vi "SSH_command.vi"(7 "password":string, 8 "error in":errorcluster, 9 "Username":string, 10 "Host":string="130.64.87.197", 11 "Command(s) to Execute":string="pwd") -> (0 "error out":errorcluster, 2 "standard error":string, 3 "standard output":string)   [LabVIEW 2012]
panel:
  out "command line input":string
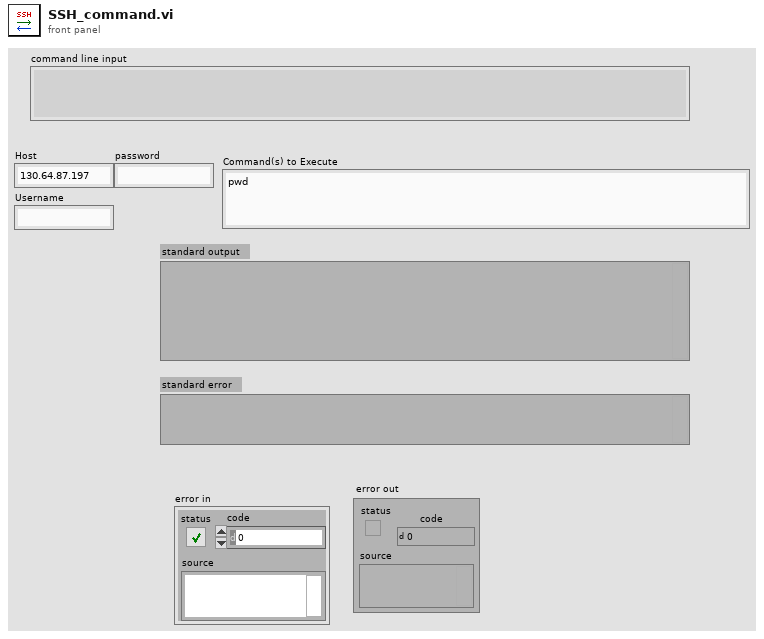
[diagram p1: front panel]
types:
  T1 = enum16{"open", "replace", "create", "open or create", "replace or create", "replace or create with confirmation"}
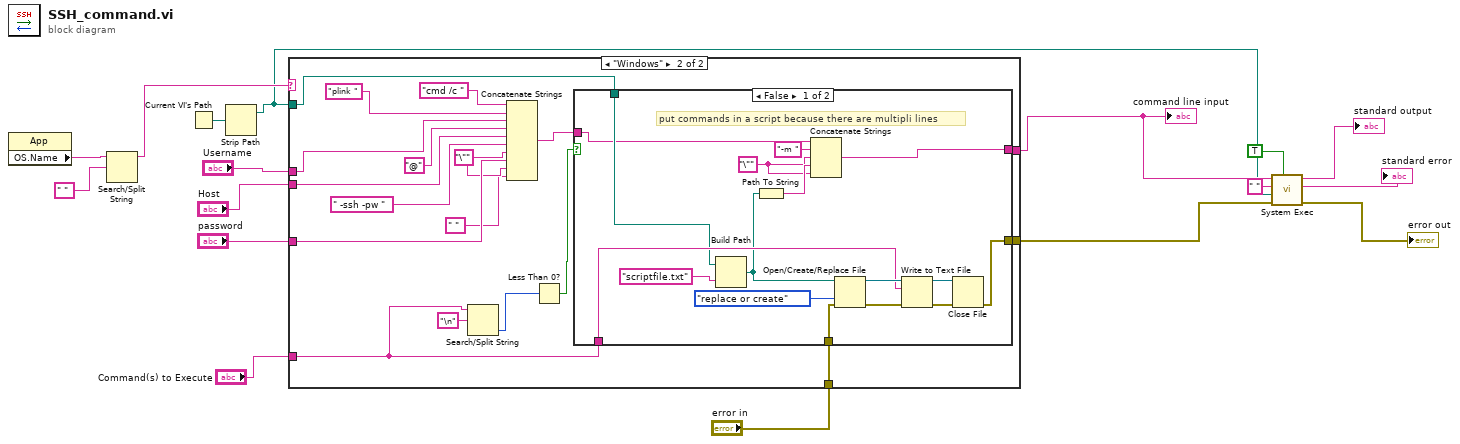
[diagram p0: block diagram]
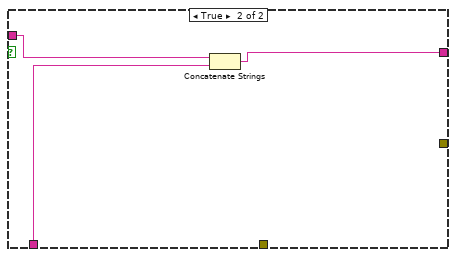
[diagram p3: hidden frame]
diagram:
  n1 = property class="App"() -> ("OS.Name"=w14:string)  [unwired: 2 in, 2 out]
  n2 = Search/Split String(string=w14, search string/char (-)=" ") -> (substring before match=w13:string)  [unwired: 1 in, 2 out]
  n3 = Current VI's Path() -> (path=w17:path)
  n4 = Strip Path(path=w17) -> (stripped path=w7:path)  [unwired: 1 out]
  n5 = case shown="\"Windows\"" w13 {
    tunnel: w7 -> [_ w30]
    tunnel: "Username" -> [_ w34]
    tunnel: "Host" -> [_ w32]
    tunnel: "password" -> [_ w27]
    tunnel: "Command(s) to Execute" -> [_ w22]
    tunnel: [_ w28] -> w10
    tunnel: [_ w19] -> w2
    tunnel: "error in" -> [_ w18]
    frame "False", Default {
    }
    frame "Windows" {
      w26 = "\"" ("string")
      n6 = Search/Split String(string=w22, search string/char (-)="\n") -> (offset of match=w21:i32)  [unwired: 1 in, 2 out]
      n7 = Concatenate Strings("cmd /c " ("string"), "plink " ("name or relative path"), w34, "@" ("string"), w32, " -ssh -pw " ("string"), w26, w27, w26, " " ("string")) -> (w29:string)
      n8 = Less Than 0?(x=w21) -> (x < 0?=w20:bool)
      n9 = case shown="False" w20 {
        tunnel: w22 -> [w46 w53]
        tunnel: w30 -> [w44 _]
        tunnel: w29 -> [w43 w54]
        tunnel: [w40 w52] -> w28
        tunnel: [w37 _] -> w19
        tunnel: w18 -> [w36 _]
        frame False {
          w38 = "\"" ("string")
          # "put commands in a script because there are multipli lines"
          n10 = Build Path(base path=w44, name or relative path="scriptfile.txt" ("Script File Name")) -> (appended path=w41:path)
          n11 = Path To String(path=w41) -> (string=w39:string)
          n12 = Concatenate Strings(w43, "-m " ("string"), w38, w39, w38) -> (w40:string)
          n13 = Open/Create/Replace File(file path (use dialog)=w41, error in=w36, operation (0:open)=T1."replace or create") -> (refnum out=w49:refnum<file>, error out=w48:errorcluster)  [unwired: 3 in, 1 out]
          n14 = Write to Text File(file (use dialog)=w49, text=w46, error in=w48) -> (refnum out=w51:refnum<file>, error out=w50:errorcluster)  [unwired: 2 out]
          n15 = Close File(refnum=w51, error in=w50) -> (error out=w37:errorcluster)  [unwired: 1 out]
        }
        frame True {
          n16 = Concatenate Strings(w54, w53) -> (w52:string)
        }
      }
    }
  }
  "command line input" <- w10
  n17 = call <vilib>:"System Exec.vi"("wait until completion? (T)"=TRUE, "error in (no error)"=w2, "working directory"=w7, "standard input"=" ", "command line"=w10) -> ("error out"=→"error out":errorcluster, "standard error"=→"standard error":string, "standard output"=→"standard output":string)  [unwired: 3 in, 1 out]
